vi "ValidatePath.vi"(8 "error constant":errorcluster, 10 "Path":path) -> (0 "error inditcator 2":errorcluster, 2 "Path":path)   [LabVIEW 2020]
uses:
  <vilib>/Utility/error.llb/Error Cluster From Error Code.vi
  <vilib>/ErrorRing/Error Ring.xnode
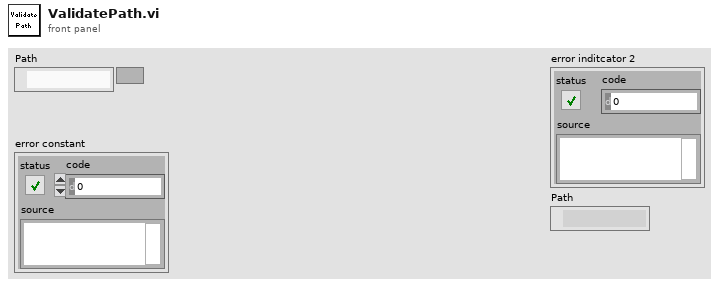
[diagram p1: front panel]
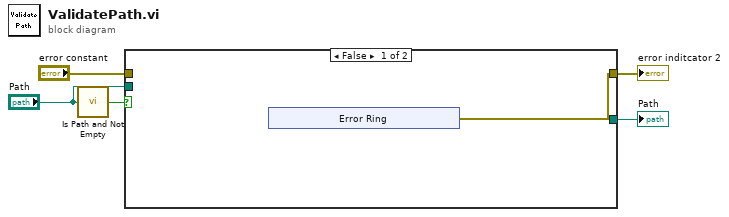
[diagram p0: block diagram]
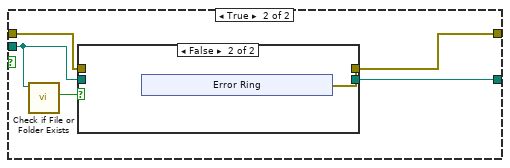
[diagram p2: hidden frame]
diagram:
  n1 = call <vilib>:"Is Path and Not Empty.vi"("path"="Path") -> ("Is Path and Not Empty?"=w2:bool)  [unwired: 4 in]
  n2 = case shown="False" w2 {
    tunnel: [w6 w16] -> w5
    tunnel: [_ w15] -> w4
    tunnel: "Path" -> [_ w14]
    tunnel: "error constant" -> [_ w12]
    frame False {
      n3 = xnode "Error Ring"() -> ("error out"=w6:errorcluster)
    }
    frame True {
      n4 = call <vilib>:"Check if File or Folder Exists.vi"("path"=w14) -> ("file or folder exists?"=w13:bool)  [unwired: 8 in, 2 out]
      n5 = case shown="False" w13 {
        tunnel: [w17 w19] -> w16
        tunnel: [w18 _] -> w15
        tunnel: w14 -> [w18 _]
        tunnel: w12 -> [w17 _]
        frame True {
        }
        frame False {
          n6 = xnode "Error Ring"() -> ("error out"=w19:errorcluster)
        }
      }
    }
  }
  "error inditcator 2" <- w5
  "Path" <- w4
